vi "Autonomous Independent.vi"() -> ()   [LabVIEW 2015]
doc: "This VI is called when autonomous begins, and will automatically be terminated when autonomous ends. You can carry out timed or sensor driven robot movement independently without needing to return to the caller."
uses:
  <vilib>/Analysis/baseanly.llb/Mean (DBL).vi
  <vilib>/Rock Robotics/WPI/Utilities/WPI_GetSetVariantRefNum.vi
  <vilib>/Rock Robotics/Network Tables/NT Write Numeric Array.vi
  <vilib>/Rock Robotics/Network Tables/NT Read Numeric Array.vi
  <vilib>/Rock Robotics/Network Tables/NT Read String Array.vi
  <vilib>/Rock Robotics/Network Tables/NT Write Number.vi
  <vilib>/Rock Robotics/WPI/RobotDrive/WPI_RobotDriveMecanumDrive_Cartesian.vi
  <vilib>/Rock Robotics/Network Tables/NT Write String.vi
  <vilib>/addons/control/pid/pid.llb/PID (DBL).vi
  <vilib>/addons/control/pid/NI_PID_pid.lvlib
  <vilib>/Analysis/NI_AALBase.lvlib
panel:
  out "Waveform Chart":dbl(graph)
  out "Rotate PID Output":dbl(graph)
  # "Be sure to right-click and choose Data Operations>>Make Current Value default if you want to save the array values with the VI"
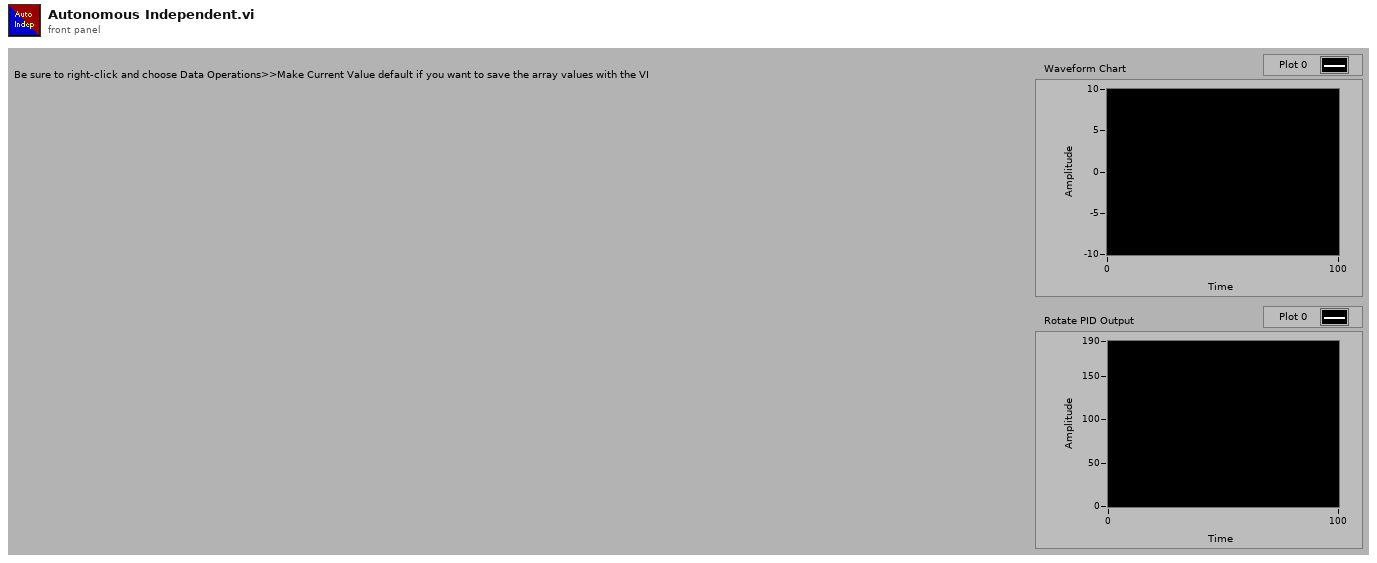
[diagram p1: front panel]
types:
  T1 = typedef "WPI_JoystickDevRef.ctl" = cluster{"Device":T2}
  T2 = typedef "WPI_JoystickDeviceEnum.ctl" = enum16{"USB 0", "USB 1", "USB 2", "USB 3", "USB 4", "USB 5"}
  T3 = typedef "WPI_EncoderDevRef.ctl" = cluster{"DevStatus":errorcluster, "EncoderIndex":T4, "CounterIndex":T5, "DistancePerCount":dbl, "Decoding Type":T6}
  T4 = typedef "FPGA_EncoderIdx.ctl" = enum8{"Enc 0", "Enc 1", "Enc 2", "Enc 3", "Enc 4", "Enc 5", "Enc 6", "Enc 7", "Invalid"}
  T5 = typedef "FPGA_CounterCtrSystemIndex.ctl" = enum8{"Ctr 0", "Ctr 1", "Ctr 2", "Ctr 3", "Ctr 4", "Ctr 5", "Ctr 6", "Ctr 7", "Invalid"}
  T6 = typedef "WPI_EncoderType.ctl" = enum16{"1x", "2x", "4x"}
  T7 = cluster{"proportional gain (Kc)":dbl, "integral time (Ti, min)":dbl, "derivative time (Td, min)":dbl}
  T8 = typedef "WPI_GyroDevRef.ctl" = cluster{"DevStatus":errorcluster, "Analog Channel":T9, "Offset":dbl, "Gain (VoltsPerDegree/Second)":dbl, "Gyro Type":enum16{"Analog", "XRS450"}, "Handle":i32, "SPI Bus":T10, "Device Found":bool, "Sample Rate":dbl, "Calibrate On Open":bool}
  T9 = typedef "FPGA_AIChannel.ctl" = enum8{"AI 0", "AI 1", "AI 2", "AI 3", "AI MXP 0", "AI MXP 1", "AI MXP 2", "AI MXP 3", "Invalid"}
  T10 = typedef "spi_bus.ctl" = enum16{"SPI On-Board, CS0", "SPI On-Board, CS1", "SPI On-Board, CS2", "SPI On-Board, CS3", "SPI MXP", "Invalid"}
  T11 = typedef "WPI_RobotDriveDevRef.ctl" = cluster{"DevStatus":errorcluster, "Motors[]":T12[], "Square Inputs":bool, "Max Output":dbl}
  T12 = typedef "WPI_MotorControlDeviceRef.ctl" = cluster{"DeviceStatus":errorcluster, "Type":T13, "PWM":cluster{"PWM Channel":T14, "DeadBand":T15}, "CAN":cluster{"Device Number":u8, "Control Mode":T16, "Semaphore":T17, "Max Vout":dbl, "TalonSRX Control Mode":T18}, "Invert":bool}
  T13 = typedef "WPI_MotorControlType.ctl" = enum16{"PWM", "CAN", "CANTalonSRX"}
  T14 = typedef "FPGA_DIOPWMChannel.ctl" = enum8{"PWM 0", "PWM 1", "PWM 2", "PWM 3", "PWM 4", "PWM 5", "PWM 6", "PWM 7", "PWM 8", "PWM 9", "PWM MXP 0", "PWM MXP 1", "PWM MXP 2", "PWM MXP 3", "PWM MXP 4", "PWM MXP 5", "PWM MXP 6", "PWM MXP 7", "PWM MXP 8", "PWM MXP 9", "Invalid"}
  T15 = typedef "WPI_PWMDeadband.ctl" = cluster{"Name":string, "maxPositivePwm":i32, "minPositivePwm":i32, "centerPwm":i32, "maxNegativePwm":i32, "minNegativePwm":i32, "angularRange":u16}
  T16 = typedef "WPI_CANJaguar_ControlMode.ctl" = enum8{"Percent VBus", "Current", "Speed", "Position", "Voltage"}
  T17 = typedef "Semaphore RefNum" = refnum<k1>
  T18 = typedef "WPI_CANTalonSRX_APIControlMode.ctl" = enum8{"Percent VBus", "Speed", "Position", "Slave", "Unchanged / Invalid", "Voltage Compensation", "Current", "Motion Profile"}
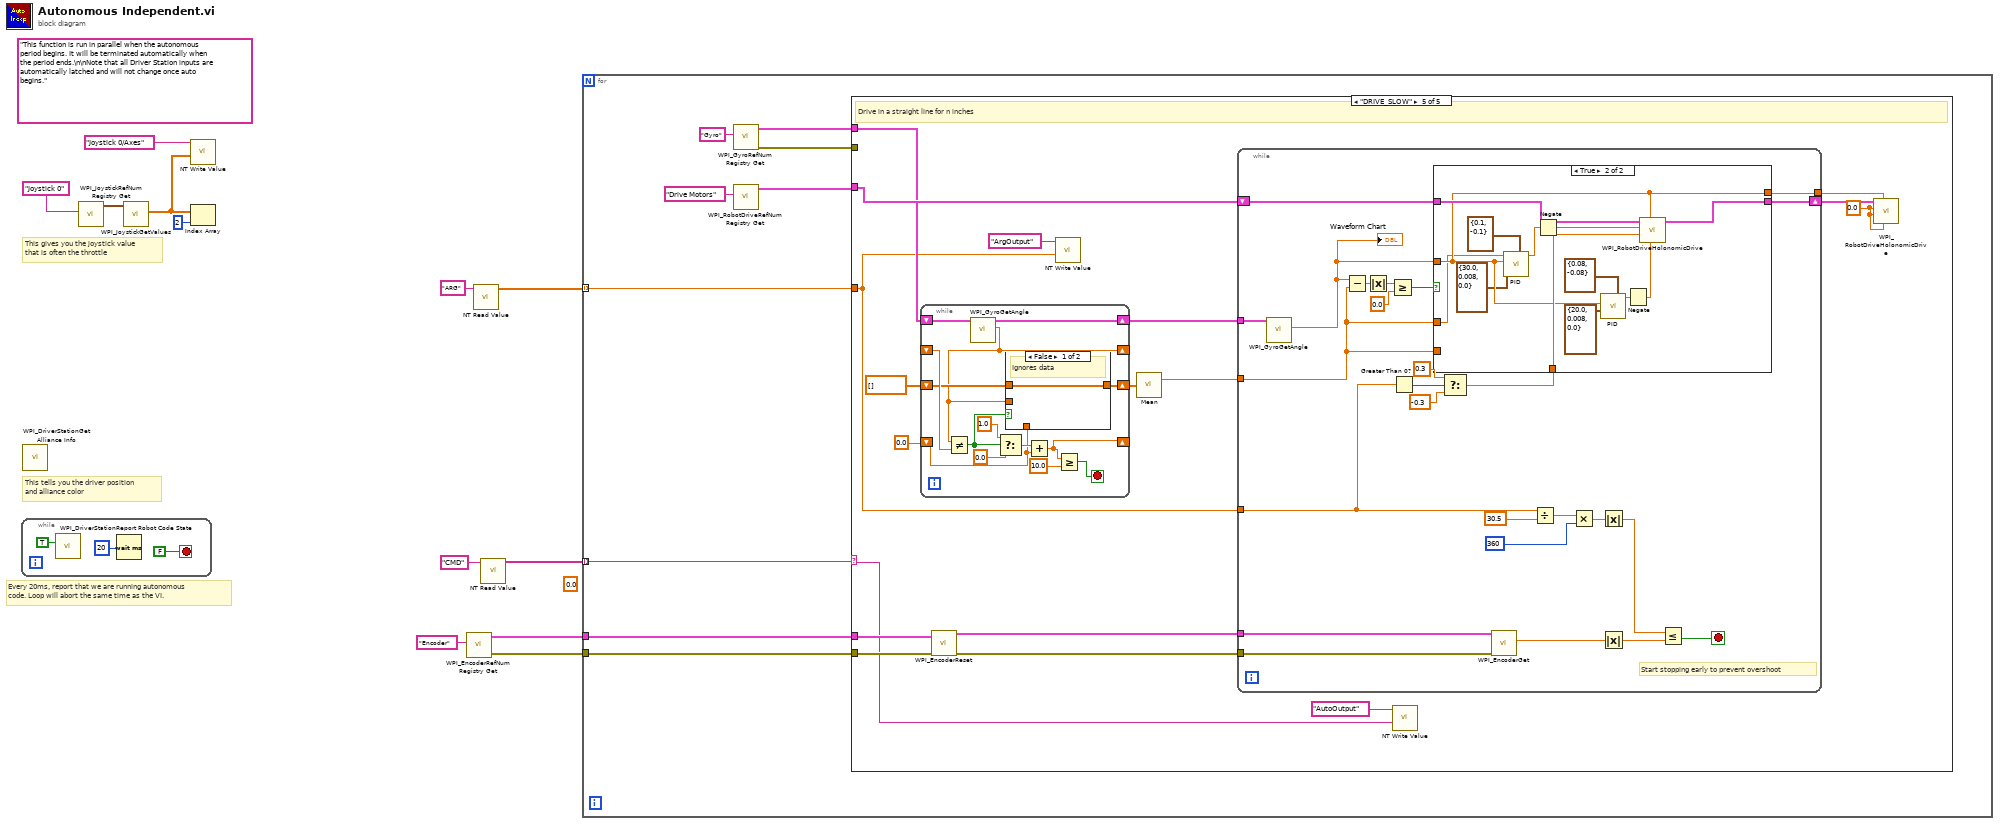
[diagram p0: block diagram]
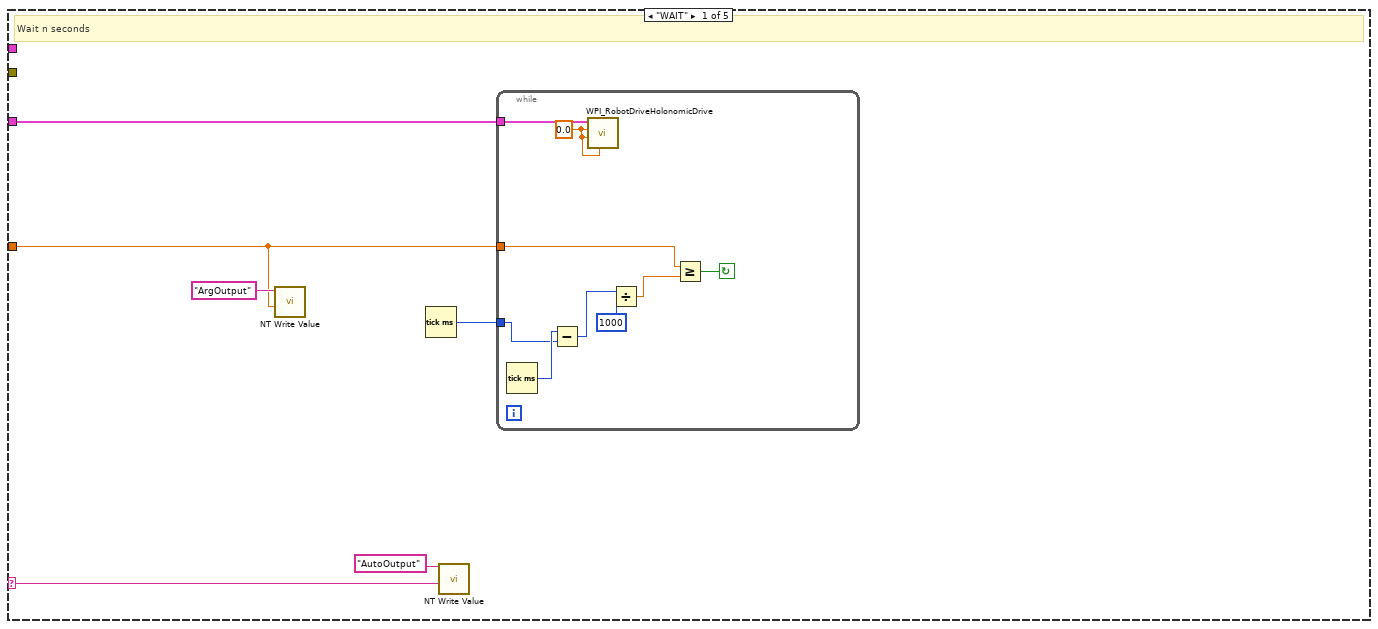
[diagram p2: hidden frame]
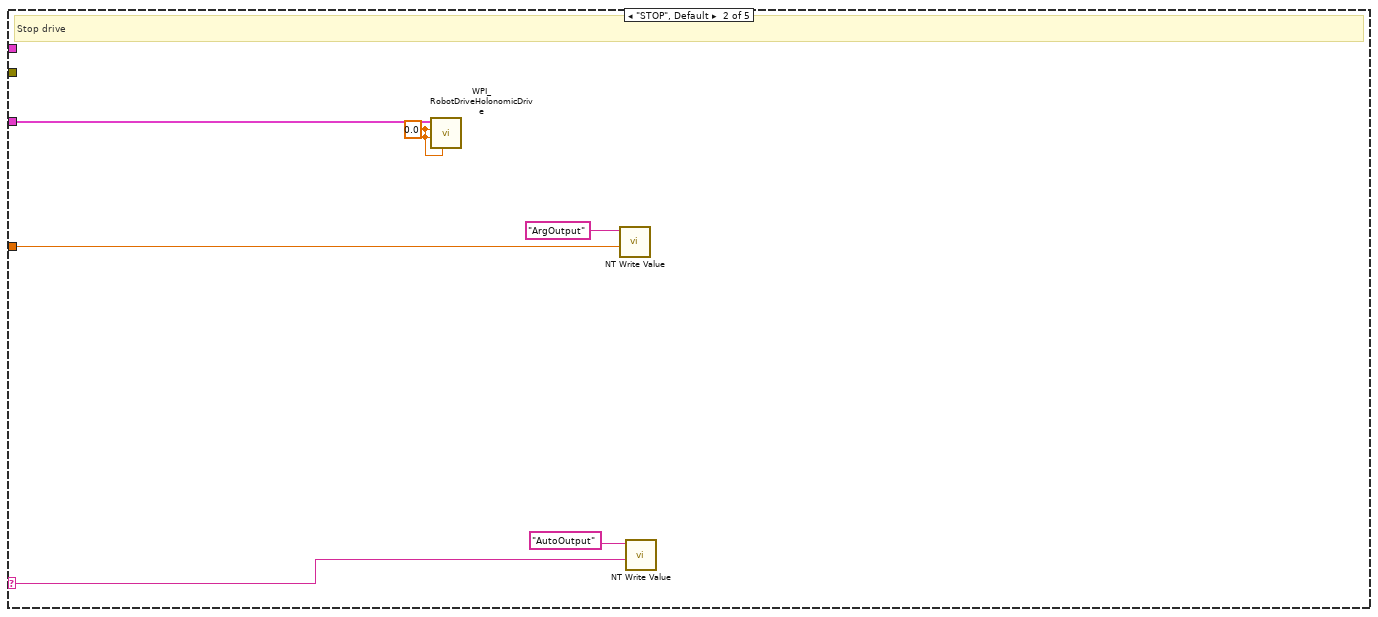
[diagram p3: hidden frame]
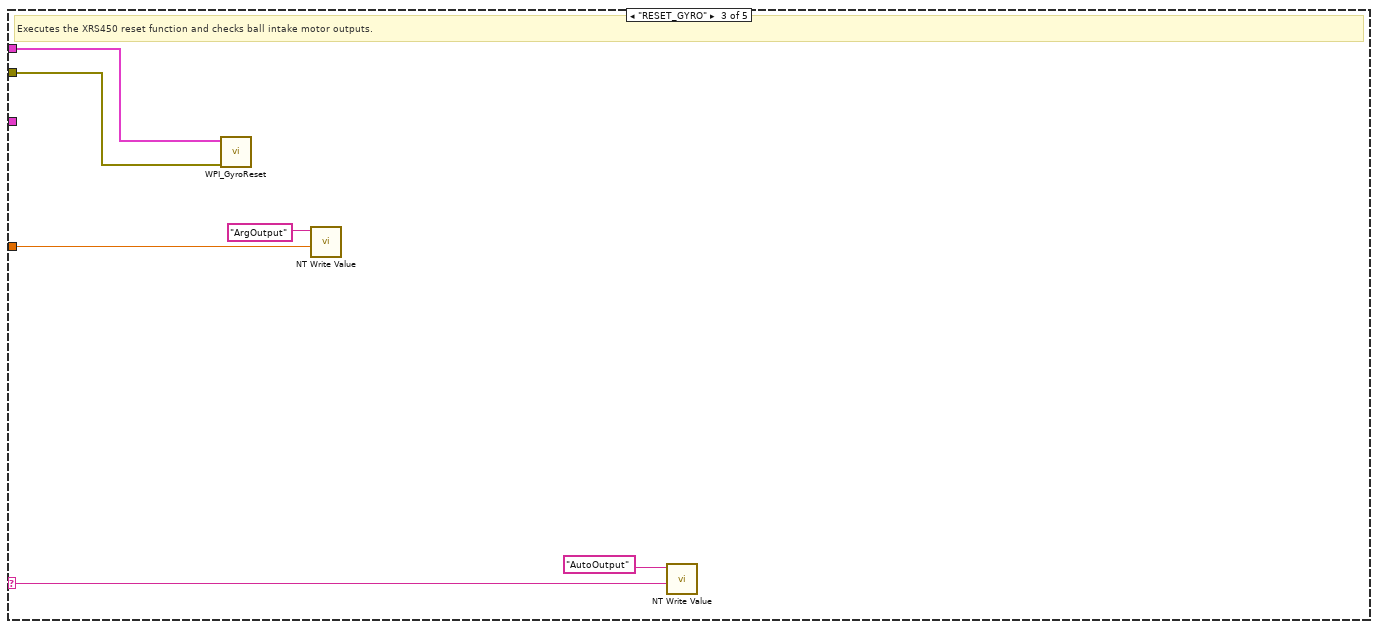
[diagram p4: hidden frame]
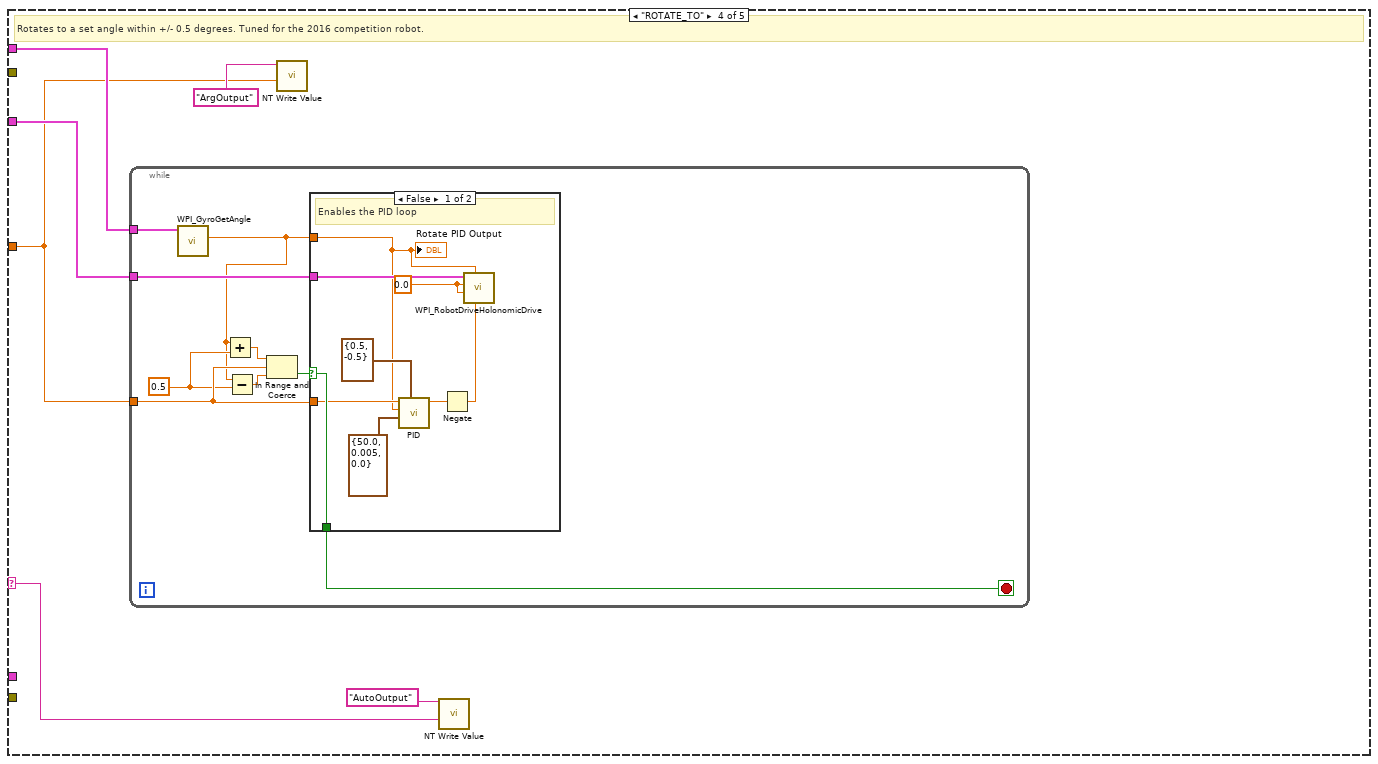
[diagram p5: hidden frame]
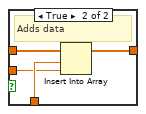
[diagram p8: hidden frame]
diagram:
  (unwired) 0.0 ("Motor Output")
  (unwired) "This function is run in parallel when the autonomous period begins. It will be terminated automatically when the period ends.\n\nNote that all Driver Station inputs are automatically latched and will not change once auto begins."
  # "Every 20ms, report that we are running autonomous\ncode. Loop will abort the same time as the VI."
  # "This gives you the joystick value\nthat is often the throttle"
  # "This tells you the driver position\nand alliance color"
  n1 = while {
    stop <- FALSE stop-if-true
    n2 = call <vilib>:"WPI_DriverStationReport Robot Code State.vi"("Autonomous"=TRUE) -> ()  [unwired: 10 in, 1 out]
    n3 = Wait (ms)(milliseconds to wait=u32 20) -> ()  [unwired: 1 out]
  }
  n4 = call <vilib>:"WPI_DriverStationGet Alliance Info.vi"() -> ()  [unwired: 12 out]
  n5 = call <vilib>:"WPI_JoystickRefNum Registry Get.vi"("refnum name"="Joystick 0") -> ("JoystickDevRef"=w11:T1)  [unwired: 1 in, 9 out]
  n6 = call <vilib>:"WPI_JoystickGetValues.vi"("JoystickDevRef"=w11) -> ("Axes"=w9:dbl[])  [unwired: 6 in, 4 out]
  n7 = call-poly <vilib>:"NT Write Value.vi"("Numeric Array"=w9, "Name"="Joystick 0/Axes") -> ()  [unwired: 9 in, 1 out]
  n8 = Index Array(array=w9, index=2) -> ()  [unwired: 1 out]
  n9 = call <vilib>:"WPI_EncoderRefNum Registry Get.vi"("refnum name"="Encoder") -> ("error out"=w1:errorcluster, "EncoderDevRef"=w2:T3)  [unwired: 9 in]
  n10 = call-poly <vilib>:"NT Read Value.vi"("Name"="ARG") -> ("Numeric Array"=w5:dbl[])  [unwired: 9 in, 1 out]
  n11 = call-poly <vilib>:"NT Read Value.vi"("Name"="CMD") -> ("String Array"=w4:string[])  [unwired: 9 in, 1 out]
  n12 = for {
    tunnel: w4 -> [w24] mode=indexing
    tunnel: w5 -> [w23] mode=indexing
    tunnel: w2 -> [w22]
    tunnel: w1 -> [w21]
    n13 = call <vilib>:"WPI_GyroRefNum Registry Get.vi"("refnum name"="Gyro") -> ("error out"=w18:errorcluster, "GyroDevRef"=w19:T8)  [unwired: 9 in]
    n14 = call <vilib>:"WPI_RobotDriveRefNum Registry Get.vi"("refnum name"="Drive Motors") -> ("RobotDriveDevRef"=w17:T11)  [unwired: 9 in, 1 out]
    n15 = case shown="\"DRIVE_SLOW\"" w24 {
      selector: w24 -> [w29 w45 w50 w56 w88]
      tunnel: w17 -> [w28 w41 _ w55 w87]
      tunnel: w23 -> [w25 w42 w46 w52 w81]
      tunnel: w22 -> [_ _ _ _ w93]
      tunnel: w21 -> [_ _ _ _ w92]
      tunnel: w19 -> [_ _ w49 w54 w83]
      tunnel: w18 -> [_ _ w48 _ _]
      frame "WAIT" {
        # "Wait n seconds"
        n16 = call-poly <vilib>:"NT Write Value.vi"("Numeric"=w25, "Name"="ArgOutput") -> ()  [unwired: 9 in, 1 out]
        n17 = Tick Count (ms)() -> (millisecond timer value=w27:u32)
        n18 = call-poly <vilib>:"NT Write Value.vi"("String"=w29, "Name"="AutoOutput") -> ()  [unwired: 9 in, 1 out]
        n19 = while {
          tunnel: w25 -> [w36]
          tunnel: w28 -> [w33]
          tunnel: w27 -> [w34]
          stop <- w31 continue-if-true
          w32 = 0.0 ("X")
          n20 = Tick Count (ms)() -> (millisecond timer value=w35:u32)
          n21 = Subtract(x=w35, y=w34) -> (x-y=w39:u32)
          n22 = call-poly <vilib>:"WPI_RobotDriveHolonomicDrive.vi"("Rotation"=w32, "Y"=w32, "X"=w32, "RobotDriveDevRef"=w33) -> ()  [unwired: 5 in, 3 out]
          n23 = Divide(x=w39, y=u32 1000) -> (x/y=w37:dbl)
          n24 = Greater Or Equal?(x=w36, y=w37) -> (x >= y?=w31:bool)
        }
      }
      frame "STOP", Default {
        w40 = 0.0 ("Y")
        # "Stop drive"
        n25 = call-poly <vilib>:"WPI_RobotDriveHolonomicDrive.vi"("Rotation"=w40, "Y"=w40, "X"=w40, "RobotDriveDevRef"=w41) -> ()  [unwired: 5 in, 3 out]
        n26 = call-poly <vilib>:"NT Write Value.vi"("Numeric"=w42, "Name"="ArgOutput") -> ()  [unwired: 9 in, 1 out]
        n27 = call-poly <vilib>:"NT Write Value.vi"("String"=w45, "Name"="AutoOutput") -> ()  [unwired: 9 in, 1 out]
      }
      frame "RESET_GYRO" {
        # "Executes the XRS450 reset function and checks ball intake motor outputs."
        n28 = call <vilib>:"WPI_GyroReset.vi"("error in"=w48, "GyroDevRef"=w49) -> ()  [unwired: 8 in, 2 out]
        n29 = call-poly <vilib>:"NT Write Value.vi"("Numeric"=w46, "Name"="ArgOutput") -> ()  [unwired: 9 in, 1 out]
        n30 = call-poly <vilib>:"NT Write Value.vi"("String"=w50, "Name"="AutoOutput") -> ()  [unwired: 9 in, 1 out]
      }
      frame "ROTATE_TO" {
        # "Rotates to a set angle within +/- 0.5 degrees. Tuned for the 2016 competition robot."
        n31 = while {
          tunnel: w52 -> [w61]
          tunnel: w55 -> [w63]
          tunnel: w54 -> [w58]
          stop <- w66 stop-if-true
          w60 = 0.5 ("Within")
          n32 = call <vilib>:"WPI_GyroGetAngle.vi"("GyroDevRef"=w58) -> ("Angle"=w59:dbl)  [unwired: 6 in, 4 out]
          n33 = Add(x=w59, y=w60) -> (x+y=w65:dbl)
          n34 = Subtract(x=w59, y=w60) -> (x-y=w64:dbl)
          n35 = In Range and Coerce(upper limit=w65, x=w61, lower limit=w64) -> (In Range?=w62:bool)  [unwired: 1 out]
          n36 = case shown="False" w62 {
            selector: w62 -> [w73 w76]
            tunnel: w61 -> [w72 _]
            tunnel: [w73 w76] -> w66
            tunnel: w59 -> [w70 _]
            tunnel: w63 -> [w71 _]
            frame False {
              w68 = 0.0 ("X")
              # "Enables the PID loop"
              n37 = call-poly <vilib>:"PID.vi"("output range"=cluster{"output high":dbl, "output low":dbl} {"output high"=0.5, "output low"=-0.5}, "PID gains"=T7 {"proportional gain (Kc)"=50.0, "integral time (Ti, min)"=0.005, "derivative time (Td, min)"=0.0}, "process variable"=w70, "setpoint"=w72) -> ("output"=w69:dbl)  [unwired: 6 in, 1 out]
              n38 = Negate(x=w69) -> (-x=w67:dbl)
              n39 = call-poly <vilib>:"WPI_RobotDriveHolonomicDrive.vi"("Rotation"=w67, "Gyro Angle"=w70, "Y"=w68, "X"=w68, "RobotDriveDevRef"=w71) -> ()  [unwired: 4 in, 3 out]
              "Rotate PID Output" <- w70
            }
            frame True {
              # "Disables the PID loop"
            }
          }
        }
        n40 = call-poly <vilib>:"NT Write Value.vi"("Numeric"=w52, "Name"="ArgOutput") -> ()  [unwired: 9 in, 1 out]
        n41 = call-poly <vilib>:"NT Write Value.vi"("String"=w56, "Name"="AutoOutput") -> ()  [unwired: 9 in, 1 out]
      }
      frame "DRIVE_SLOW" {
        w78 = 0.0 ("X")
        # "Drive in a straight line for n inches"
        n42 = while {
          shift-right: [w137] -> _
          shift-left: _ -> [w148]
          shift-right: [w140] -> _
          shift-left: 0.0 -> [w138]
          shift-right: [w135] -> w86
          shift-left: w83 -> [w136]
          shift-right: [w139] -> w90
          shift-left: dbl[] [] -> [w141]
          stop <- w144 stop-if-true
          n43 = call <vilib>:"WPI_GyroGetAngle.vi"("GyroDevRef"=w136) -> ("Angle"=w137:dbl, "GyroDevRef"=w135:T8)  [unwired: 6 in, 3 out]
          n44 = Not Equal?(x=w137, y=w148) -> (x != y?=w142:bool)
          n45 = Select(t=1.0, s=w142, f=0.0) -> (s? t:f=w145:dbl)
          n46 = case shown="False" w142 {
            tunnel: w141 -> [w149 w153]
            tunnel: [w149 w152] -> w139
            tunnel: w137 -> [_ w150]
            tunnel: w138 -> [_ w151]
            frame False {
              # "Ignores data"
            }
            frame True {
              # "Adds data"
              n47 = Insert Into Array(array=w153, index=w151, new element=w150) -> (w152:dbl[])
            }
          }
          n48 = Add(x=w145, y=w138) -> (x+y=w140:dbl)
          n49 = Greater Or Equal?(x=w140, y=10.0) -> (x >= y?=w144:bool)
        }
        n50 = call <vilib>:"WPI_EncoderReset.vi"("error in (no error)"=w92, "EncoderDevRef"=w93) -> ("error out"=w84:errorcluster, "EncoderDevRef"=w85:T3)  [unwired: 8 in]
        n51 = call-poly <vilib>:"NT Write Value.vi"("Numeric"=w81, "Name"="ArgOutput") -> ()  [unwired: 9 in, 1 out]
        n52 = call-poly <vilib>:"Mean.vi"("X"=w90) -> ("mean"=w77:dbl)  [unwired: 1 out]
        n53 = while {
          tunnel: w86 -> [w100]
          tunnel: w77 -> [w98]
          shift-right: [w119] -> w80
          shift-left: w87 -> [w118]
          tunnel: w81 -> [w102]
          tunnel: w85 -> [w110]
          tunnel: w84 -> [w109]
          tunnel: [w99] -> w79
          stop <- w111 stop-if-true
          # "Start stopping early to prevent overshoot"
          n54 = call <vilib>:"WPI_GyroGetAngle.vi"("GyroDevRef"=w100) -> ("Angle"=w101:dbl)  [unwired: 6 in, 4 out]
          "Waveform Chart" <- w101
          n55 = Subtract(x=w101, y=w98) -> (x-y=w116:dbl)
          n56 = Absolute Value(x=w116) -> (abs(x)=w115:dbl)
          n57 = Greater Or Equal?(x=w115, y=0.0) -> (x >= y?=w103:bool)
          n58 = Greater Than 0?(x=w102) -> (x > 0?=w107:bool)
          n59 = Select(t=0.3, s=w107, f=-0.3) -> (s? t:f=w104:dbl)
          n60 = case shown="True" w103 {
            tunnel: [w121 w132] -> w119
            tunnel: w118 -> [w121 w133]
            tunnel: w101 -> [w120 w129]
            tunnel: w98 -> [_ w127]
            tunnel: w104 -> [_ w131]
            tunnel: [w120 w129] -> w99
            tunnel: w98 -> [_ _]
            frame False {
            }
            frame True {
              n61 = call-poly <vilib>:"PID.vi"("output range"=cluster{"output high":dbl, "output low":dbl} {"output high"=0.1, "output low"=-0.1}, "PID gains"=T7 {"proportional gain (Kc)"=30.0, "integral time (Ti, min)"=0.008, "derivative time (Td, min)"=0.0}, "process variable"=w129, "setpoint"=w127) -> ("output"=w124:dbl)  [unwired: 6 in, 1 out]
              n62 = Negate(x=w124) -> (-x=w123:dbl)
              n63 = call-poly <vilib>:"PID.vi"("output range"=cluster{"output high":dbl, "output low":dbl} {"output high"=0.08, "output low"=-0.08}, "PID gains"=T7 {"proportional gain (Kc)"=20.0, "integral time (Ti, min)"=0.008, "derivative time (Td, min)"=0.0}, "process variable"=w129) -> ("output"=w128:dbl)  [unwired: 7 in, 1 out]
              n64 = Negate(x=w128) -> (-x=w126:dbl)
              n65 = call-poly <vilib>:"WPI_RobotDriveHolonomicDrive.vi"("Rotation"=w126, "Gyro Angle"=w129, "Y"=w131, "X"=w123, "RobotDriveDevRef"=w133) -> ("RobotDriveDevRef"=w132:T11)  [unwired: 4 in, 2 out]
            }
          }
          n66 = call <vilib>:"WPI_EncoderGet.vi"("error in (no error)"=w109, "EncoderDevRef"=w110) -> ("Distance"=w97:dbl)  [unwired: 4 in, 5 out]
          n67 = Divide(x=w102, y=30.5) -> (x/y=w113:dbl)
          n68 = Multiply(x=w113, y=360) -> (x*y=w108:dbl)
          n69 = Absolute Value(x=w108) -> (abs(x)=w95:dbl)
          n70 = Absolute Value(x=w97) -> (abs(x)=w96:dbl)
          n71 = Less Or Equal?(x=w95, y=w96) -> (x <= y?=w111:bool)
        }
        n72 = call-poly <vilib>:"NT Write Value.vi"("String"=w88, "Name"="AutoOutput") -> ()  [unwired: 9 in, 1 out]
        n73 = call-poly <vilib>:"WPI_RobotDriveHolonomicDrive.vi"("Rotation"=w78, "Gyro Angle"=w79, "Y"=w78, "X"=w78, "RobotDriveDevRef"=w80) -> ()  [unwired: 4 in, 3 out]
      }
    }
  }
